vi "Get Installed Components.vi"(8 "error in (no error)":errorcluster, 9 "Cached (F)":bool, 10 "Item Types (all visible)":T3 items=["all visible", "all including hidden", "standard only", "startup only"], 11 "Session in":refnum<k21>) -> (0 "error out":errorcluster, 2 "Software Components":T1[](array[typedef]) {"component type" items=["standard", "hidden", "system", "unknown", "startup", "image", "essential"]}, 3 "Session out":refnum<k21>)   [LabVIEW 2017, in "nisyscfg.lvlib"]
doc: "Retrieves a list of software components installed on a Real-Time or Windows system."
uses:
  <vilib>/nisyscfg/nisyscfg.lvlib
  <vilib>/nisyscfg/Component Types.ctl
  <vilib>/nisyscfg/Software 1.2.ctl
  <vilib>/nisyscfg/Component Type.ctl
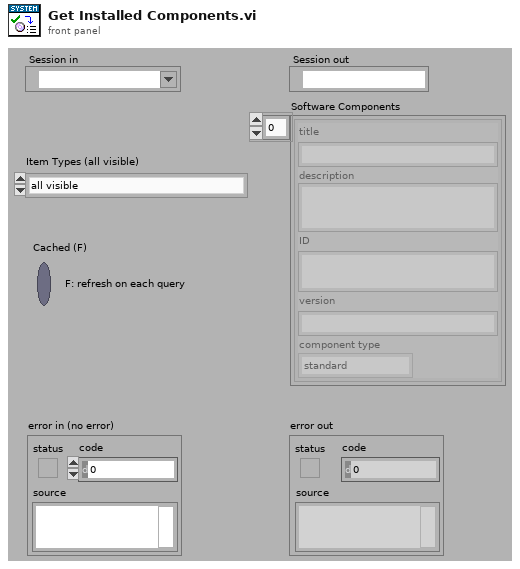
[diagram p1: front panel]
types:
  T1 = typedef "nisyscfg.lvlib/Software 1.2.ctl" = cluster{"title":string, "description":string, "ID":string, "version":string, "component type":T2}
  T2 = typedef "nisyscfg.lvlib/Component Type.ctl" = u32
  T3 = typedef "nisyscfg.lvlib/Component Types.ctl" = u32
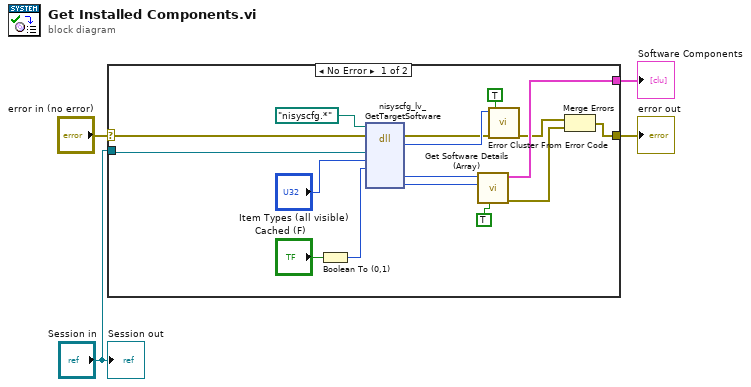
[diagram p0: block diagram]
diagram:
  n1 = case shown="No Error" "error in (no error)" {
    selector: "error in (no error)" -> [w17 w21]
    tunnel: [w9 _] -> w4
    tunnel: [w8 w21] -> w3
    tunnel: "Session in" -> [w16 _]
    frame No Error {
      n2 = Boolean To (0,1)(Boolean="Cached (F)") -> (0, 1=w18:i16)
      n3 = dll-call lib="nisyscfg.*" fn="nisyscfg_lv_GetTargetSoftware" label="GetTargetSoftware"(path in=path "nisyscfg.*", error in=w17, "system"=w16, "includeTypes"="Item Types (all visible)", "cached"=w18) -> (error out=w7:errorcluster, "result"=w20:i32, "components"=w13:u64, "numComponents"=w12:i32)  [unwired: 6 in, 1 out]
      n4 = call <vilib>:"Get Software Details (Array).vi"("Trace Component Info (F)"=TRUE ("log to NI Spy (F)"), "Number of Elements"=w12, "Enumerator in"=w13) -> ("error out"=w5:errorcluster, "Software Components"=w9:T1[])  [unwired: 7 in]
      n5 = call <vilib>:"Error Cluster From Error Code.vi"("show call chain? (False)"=TRUE, "error in (no error)"=w7, "error code (0)"=w20) -> ("error out"=w6:errorcluster)  [unwired: 6 in]
      n6 = Merge Errors(w6, w5) -> (w8:errorcluster)
    }
    frame Error {
    }
  }
  "error out" <- w3
  "Software Components" <- w4
  "Session out" <- "Session in"
